vi "RCM Show Message Log MHLC.vi"(8 "error in (no error)":errorcluster, 10 "Tree RCM Data":T1, 11 "AppMgr in":refnum<class "Application Manager.lvclass">) -> (0 "error out":errorcluster, 3 "AppMgr out":refnum<class "Application Manager.lvclass">)   [LabVIEW 2017, in "Application Manager.lvclass"]
doc: "Send Response message to open the Message Log for the selected Worker"
uses:
  Application Manager.lvclass
  Tree Right Click Menu Data.ctl
  <vilib>/Utility/miscctls.llb/LVPoint32TypeDef.ctl
  Application Manager.lvclass/Application Manager.ctl
  rsp_Show Message Log.ctl
  Common VIs/DC_UID.ctl
  <vilib>/Utility/error.llb/Error Cluster From Error Code.vi
  <vilib>/ErrorRing/Error Ring.xnode
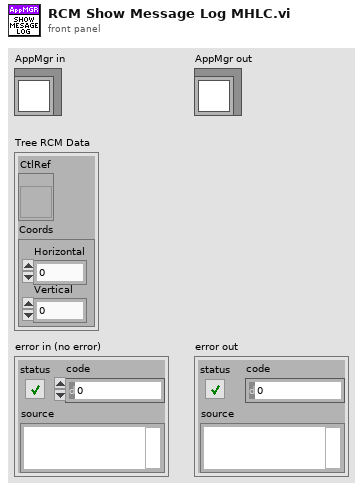
[diagram p1: front panel]
types:
  T1 = typedef "Application Manager.lvclass/Tree Right Click Menu Data.ctl" = cluster{"CtlRef":refnum<vi>, "Coords":T2}
  T2 = typedef "LVPoint32TypeDef.ctl" = cluster{"Horizontal":i32, "Vertical":i32}
  T3 = typedef "DC_UID.ctl" = string
  T4 = typedef "Application Manager.lvclass/Debug Client Data.ctl" = cluster{"DC_UID":T3, "IP Address":string, "Worker Data":T5[], "Connected":bool}
  T5 = typedef "Application Manager.lvclass/Worker Data.ctl" = cluster{"ID":string, "VI Ref":refnum<vi>, "VI Path":path, "CloneID":string, "Type":T6, "Worker Status":string}
  T6 = typedef "Workers.lvlib/Worker.lvclass/Worker Type.ctl" = enum16{"SL", "DL"}
  T7 = typedef "Application Manager.lvclass/rsp_Show Message Log.ctl" = cluster{"DC_UID":T3, "Head Worker ID":string, "IP Address":string}
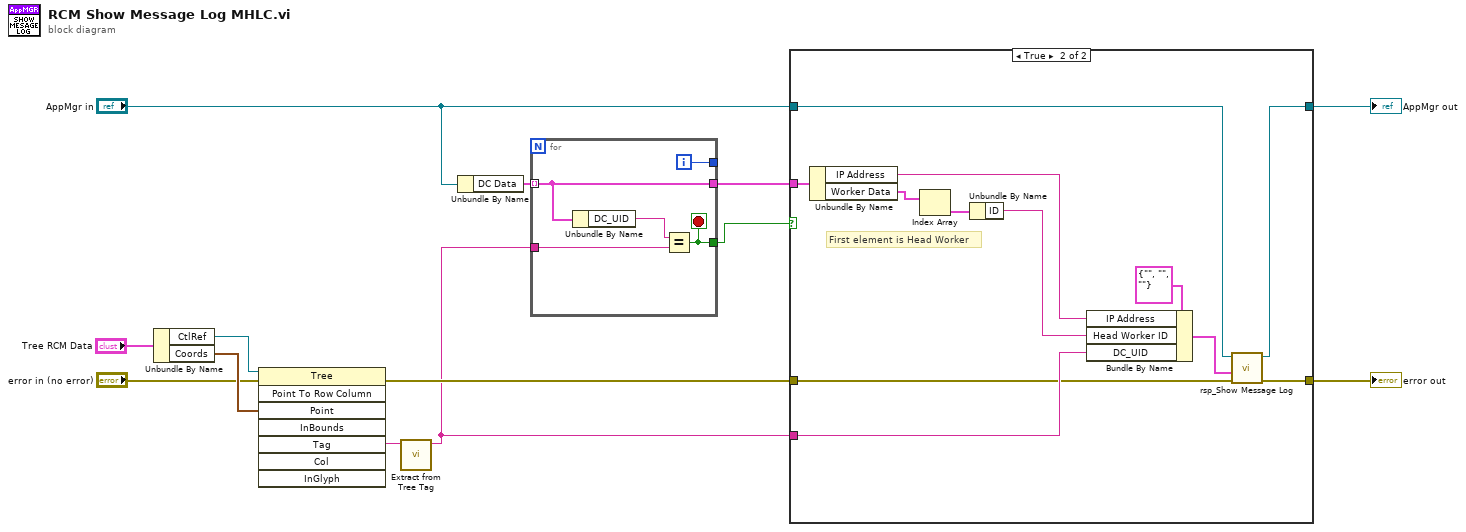
[diagram p0: block diagram]
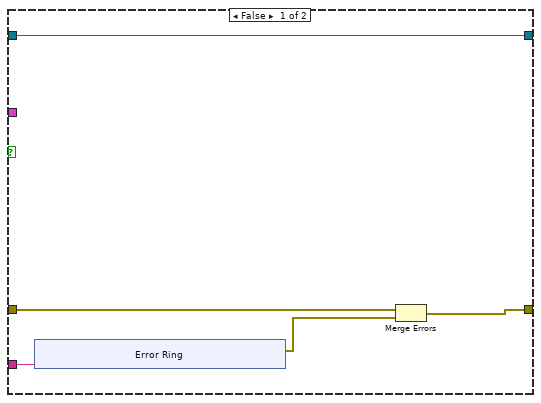
[diagram p2: hidden frame]
diagram:
  n1 = Unbundle By Name("Tree RCM Data") -> ("CtlRef"=w10:refnum<vi>, "Coords"=w9:T2)
  n2 = invoke class="Tree" method="Point To Row Column"(reference=w10, error in="error in (no error)", "Point"=w9) -> (error out=w8:errorcluster, "Tag"=w7:string)  [unwired: 5 in, 6 out]
  n3 = call "Extract from Tree Tag.vi"("Tag"=w7) -> ("DC_UID"=w6:T3)  [unwired: 9 in, 1 out]
  n4 = Unbundle By Name("AppMgr in") -> ("DC Data"=w5:T4[])
  n5 = for {
    tunnel: w5 -> [w15] mode=indexing
    tunnel: [w17] -> w3
    tunnel: [w16] -> _
    tunnel: [w15] -> w4
    tunnel: w6 -> [w14]
    i -> [w16]
    stop <- w17 stop-if-true
    n6 = Unbundle By Name(w15) -> ("DC_UID"=w18:T3)
    n7 = Equal?(x=w18, y=w14) -> (x = y?=w17:bool)
  }
  n8 = case shown="True" w3 {
    tunnel: [w22 w34] -> w11
    tunnel: w8 -> [w23 w35]
    tunnel: w6 -> [w20 w37]
    tunnel: w4 -> [_ w42]
    tunnel: "AppMgr in" -> [w19 w39]
    tunnel: [w19 w38] -> w12
    frame False {
      n9 = xnode "Error Ring"("parameter 0"=w20) -> ("error out"=w21:errorcluster)
      n10 = Merge Errors(w23, w21) -> (w22:errorcluster)
    }
    frame True {
      # "First element is Head Worker"
      n11 = Unbundle By Name(w42) -> ("IP Address"=w36:string, "Worker Data"=w33:T5[])
      n12 = Index Array(array=w33) -> (element=w32:T5)  [unwired: 1 in]
      n13 = Unbundle By Name(w32) -> ("ID"=w31:string)
      n14 = Bundle By Name(cluster=T7 {"DC_UID"="", "Head Worker ID"="", "IP Address"=""} ("Data in"), "IP Address"=w36, "Head Worker ID"=w31, "DC_UID"=w37) -> (w41:T7)
      n15 = call "rsp_Show Message Log.vi"("error in"=w35, "Data in"=w41, "Application Manager in"=w39) -> ("error out"=w34:errorcluster, "dup Application Manager out"=w38:refnum<class "Application Manager.lvclass">)  [unwired: 7 in]
    }
  }
  "AppMgr out" <- w12
  "error out" <- w11
